vi "initLogdata.vi"() -> (4 "straightPath":path, 6 "ellipsePath":path, 8 "wpPath":path, 10 "dpPath":path, 15 "eta_iPath":path)   [LabVIEW 2014]
uses:
  <vilib>/imath/engines/lvmath/Plug In/_Char/NIMS_CH_character datatype.ctl
  <vilib>/imath/engines/lvmath/Plug In/_Char/NIMS_CH_String to Character Array.vi
  <vilib>/imath/engines/lvmath2/RunTimeEngine/IndexRead/NIMS V(R2).vi
  <instcachedir>/0/NIMS V(R2)_C76619605A0E4E9F8B2FA9389712AC47.lvgen/NIMS V(R2)_C76619605A0E4E9F8B2FA9389712AC47_002.vi
  <vilib>/imath/engines/lvmath/Plug In/_Char/NIMS_CH_Character 2D to String 1D.vi
  <vilib>/imath/engines/lvmath2/RunTimeEngine/BuiltInFunctions/strconcat/NIMS_strconcat.vi
  <vilib>/imath/engines/lvmath/Plug In/_Char/NIMS_CH_String CV to Character 2D.vi
  <instcachedir>/0/NIMS_CH_String CV to Character 2D_8FC62B58B151449996F73DDB1FFD6ECB.lvgen/NIMS_CH_String CV to Character 2D_8FC62B58B151449996F73DDB1FFD6ECB_000.vi
  <vilib>/imath/engines/lvmath2/RunTimeEngine/ErrorHandling/NIMS_Create Error From Enums.vi
  <vilib>/imathl/engines/lvmath/Functions/Error Handling/Create Error.vi
  <vilib>/imath/engines/lvmath2/RunTimeEngine/NodeEndStatement/NIMS_NodeEndStatement_Output.vi
  <instcachedir>/0/NIMS_NodeEndStatement_Output_53EC0D466D134D7ABD903AC30B43404B.lvgen/NIMS_NodeEndStatement_Output_53EC0D466D134D7ABD903AC30B43404B_008.vi
  <vilib>/imath/engines/lvmath2/RunTimeEngine/ErrorHandling/NIMS_Finalize Error.vi
  <vilib>/Utility/file.llb/Write To Spreadsheet File (string).vi
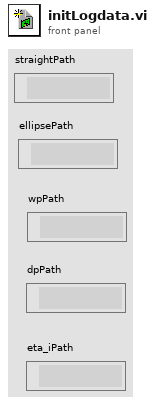
[diagram p1: front panel]
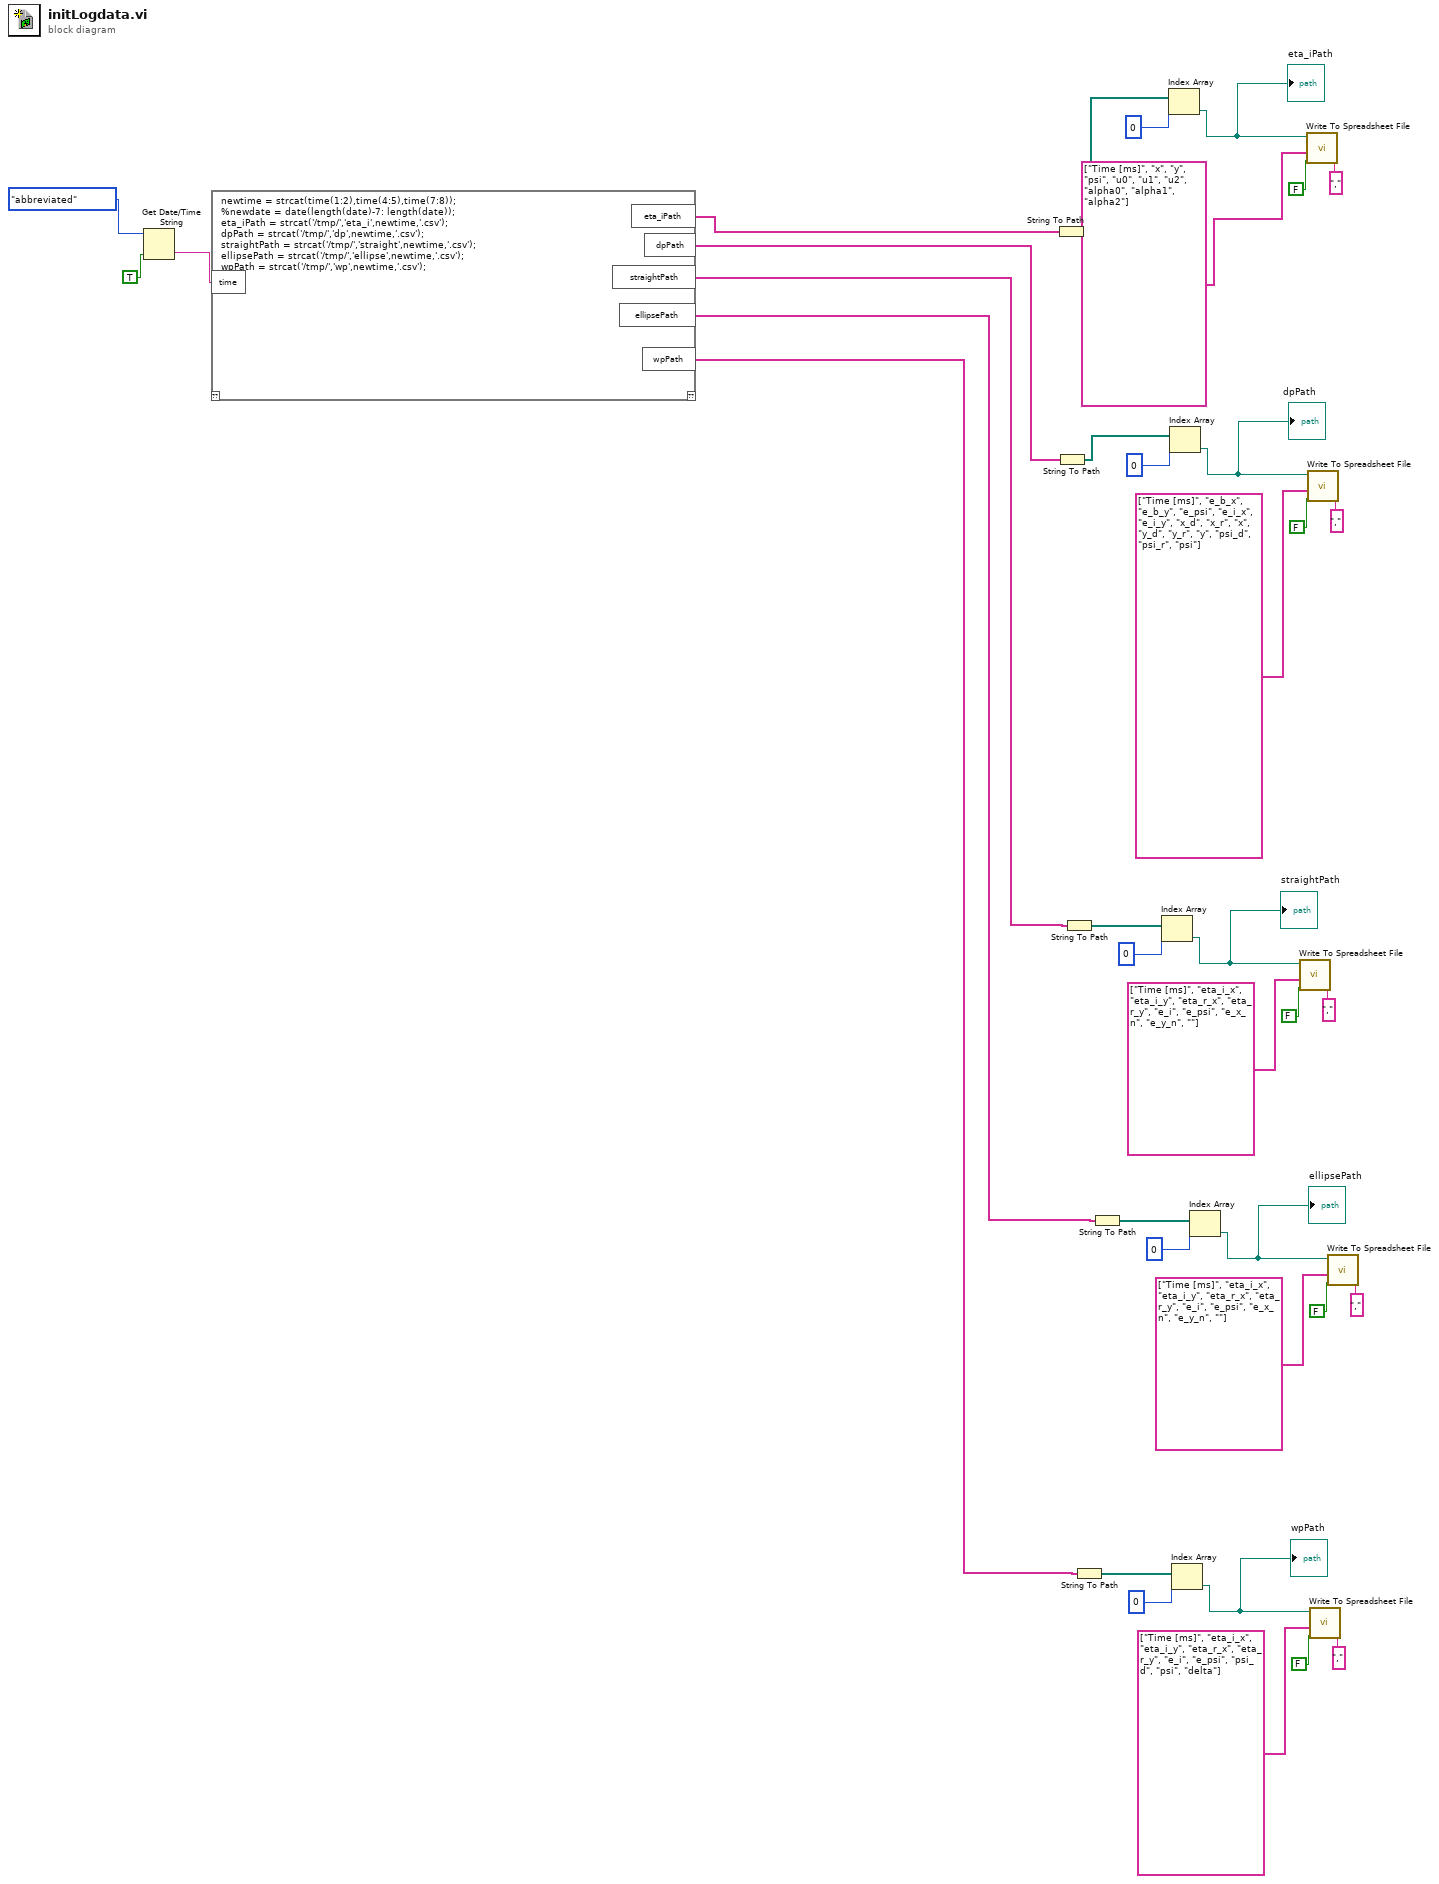
[diagram p0: block diagram]
diagram:
  n1 = Get Date/Time String(date format (0)=enum16{"short", "long", "abbreviated"}."abbreviated", want seconds? (F)=TRUE) -> (time string=w34:string)  [unwired: 1 in, 1 out]
  n2 = mathscript code="newtime = strcat(time(1:2),time(4:5),time(7:8));\n%newdate = date(length(date)-7: length(date));\neta_iPath = strcat('/tmp/','eta_i',newtime,'.csv');\ndpPath = strcat('/tmp/','dp',newtime,'.csv');\nstraightPath = strcat('/tmp/','straight',newtime,'.csv');\nellipsePath = strcat('/tmp/','ellipse',newtime,'.csv');\nwpPath = strcat('/tmp/','wp',newtime,'.csv');"("time"=w34) -> ("eta_iPath"=w24:string[], "dpPath"=w23:string[], "straightPath"=w16:string[], "ellipsePath"=w2:string[], "wpPath"=w1:string[])  [unwired: 1 in, 1 out]
  n3 = String To Path(string=w24) -> (path=w32:path[])
  n4 = String To Path(string=w23) -> (path=w26:path[])
  n5 = String To Path(string=w16) -> (path=w17:path[])
  n6 = String To Path(string=w1) -> (path=w3:path[])
  n7 = String To Path(string=w2) -> (path=w9:path[])
  n8 = Index Array(array=w17, index=0) -> (element=w18:path)
  "straightPath" <- w18
  n9 = Index Array(array=w32, index=0) -> (element=w31:path)
  "eta_iPath" <- w31
  n10 = Index Array(array=w26, index=0) -> (element=w25:path)
  "dpPath" <- w25
  n11 = Index Array(array=w3, index=0) -> (element=w4:path)
  "wpPath" <- w4
  n12 = Index Array(array=w9, index=0) -> (element=w10:path)
  "ellipsePath" <- w10
  n13 = call-poly <vilib>:"Write To Spreadsheet File.vi"("delimiter (\\t)"="," ("delimiter (\\t)"), "append to file? (new file:F)"=FALSE, "1D data"=string[] ["Time [ms]", "eta_i_x", "eta_i_y", "eta_r_x", "eta_r_y", "e_i", "e_psi", "e_x_n", "e_y_n", ""], "file path (dialog if empty)"=w18) -> ()  [unwired: 4 in, 1 out]
  n14 = call-poly <vilib>:"Write To Spreadsheet File.vi"("delimiter (\\t)"="," ("delimiter (\\t)"), "append to file? (new file:F)"=FALSE, "1D data"=string[] ["Time [ms]", "x", "y", "psi", "u0", "u1", "u2", "alpha0", "alpha1", "alpha2"], "file path (dialog if empty)"=w31) -> ()  [unwired: 4 in, 1 out]
  n15 = call-poly <vilib>:"Write To Spreadsheet File.vi"("delimiter (\\t)"="," ("delimiter (\\t)"), "append to file? (new file:F)"=FALSE, "1D data"=string[] ["Time [ms]", "e_b_x", "e_b_y", "e_psi", "e_i_x", "e_i_y", "x_d", "x_r", "x", "y_d", "y_r", "y", "psi_d", "psi_r", "psi"], "file path (dialog if empty)"=w25) -> ()  [unwired: 4 in, 1 out]
  n16 = call-poly <vilib>:"Write To Spreadsheet File.vi"("delimiter (\\t)"="," ("delimiter (\\t)"), "append to file? (new file:F)"=FALSE, "1D data"=string[] ["Time [ms]", "eta_i_x", "eta_i_y", "eta_r_x", "eta_r_y", "e_i", "e_psi", "psi_d", "psi", "delta"], "file path (dialog if empty)"=w4) -> ()  [unwired: 4 in, 1 out]
  n17 = call-poly <vilib>:"Write To Spreadsheet File.vi"("delimiter (\\t)"="," ("delimiter (\\t)"), "append to file? (new file:F)"=FALSE, "1D data"=string[] ["Time [ms]", "eta_i_x", "eta_i_y", "eta_r_x", "eta_r_y", "e_i", "e_psi", "e_x_n", "e_y_n", ""], "file path (dialog if empty)"=w10) -> ()  [unwired: 4 in, 1 out]
